vi "sendSSR.vi"(8 "error in (no error)":errorcluster, 11 "ILC in":refnum<class "ILC.lvclass">) -> (0 "error out":errorcluster, 3 "ILC out":refnum<class "ILC.lvclass">)   [LabVIEW 2015, in "ILCCommon.lvlib" / "ILC.lvclass"]
uses:
  <userlib>/Common/ILC/ILC/ILC.lvclass
  <userlib>/Common/ILC/ILC/ILC.lvclass/ILC.ctl
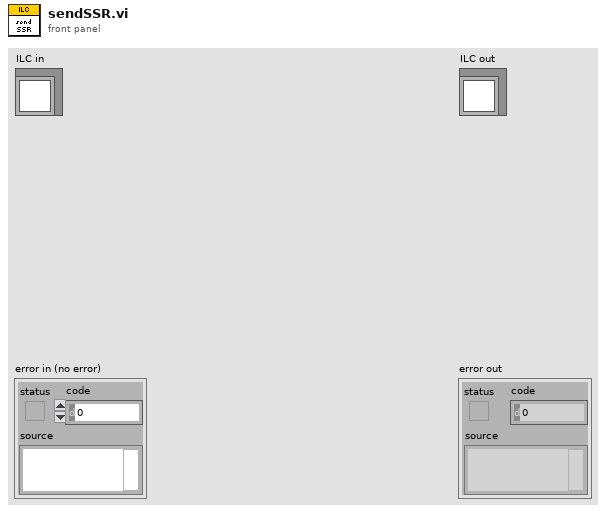
[diagram p1: front panel]
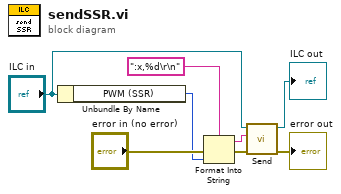
[diagram p0: block diagram]
diagram:
  n1 = Unbundle By Name("ILC in") -> ("PWM (SSR)"=w3:u8)
  n2 = Format Into String(format string=":x,%d\r\n", error in="error in (no error)", w3) -> (resulting string=w6:string, error out=w5:errorcluster)  [unwired: 1 in]
  n3 = call-dynamic "Send.vi"("error in (no error)"=w5, "Message"=w6, "ILC in"="ILC in") -> ("error out"=→"error out":errorcluster, "ILC out"=→"ILC out":refnum<class "ILC.lvclass">)  [unwired: 7 in]
